vi "Construct Raw B-Scan.vi"(0 "1D Raw Data In":u16[](array[numeric]), 1 "Resample Array":i32[](array[numeric]), 2 "B-Scan Processed In":u32, 5 "B-Scans Per Transfer":u32, 9 "A-Scans Per B-Scan":u32, 11 "Points Per A-Scan":u32, 12 "Start Trim":u32, 13 "Stop Trim":u32, 14 "Scanning Parameters":T1={"Fast Axis Offset"=0.0, "Slow Axis Offset"=0.0, "Slow Axis Amp"=4.0, "Fast Axis Amp"=4.0, "Scan Pattern"=enum."Triangle Raster"} {"Fast Axis Amp" max=20 format="%#.2f"; "Slow Axis Amp" max=20 format="%#.2f"; "Slow Axis Offset" max=10 format="%#.2f"; "Fast Axis Offset" max=10 format="%#.2f"}) -> (3 "B-Scan Processed Out":u32, 4 "B-Scan In":u16[][][](array[numeric]), 10 "A-Scan Size":i32)   [LabVIEW 2015, in "Intensity Processing.lvclass"]
uses:
  Intensity/Intensity Processing.lvclass
  Galvo/Scanning Cluster.ctl
  Galvo/Galvo.lvclass
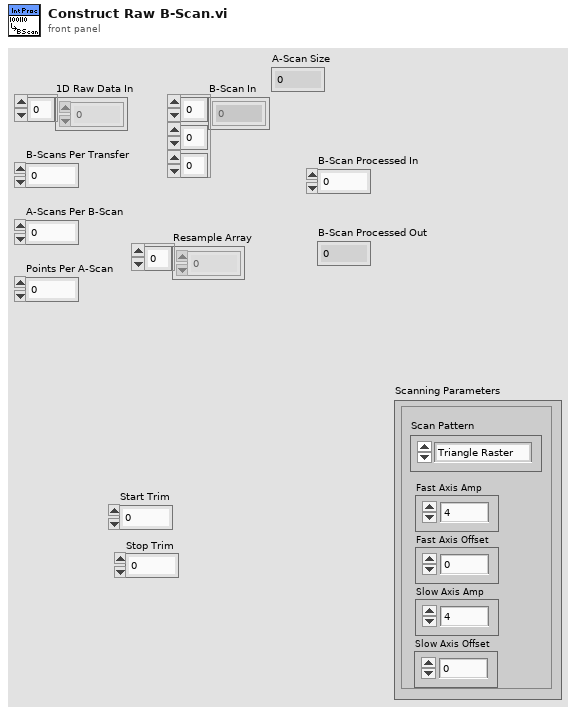
[diagram p1: front panel]
types:
  T1 = typedef "Galvo.lvclass/Scanning Cluster.ctl" = cluster{"Fast Axis Offset":sgl, "Slow Axis Offset":sgl, "Slow Axis Amp":sgl, "Fast Axis Amp":sgl, "Scan Pattern":enum16{"Raster", "Triangle Raster", "Sinusoid Raster"}}
  T2 = enum16{"Raster", "Triangle Raster", "Sinusoid Raster"}
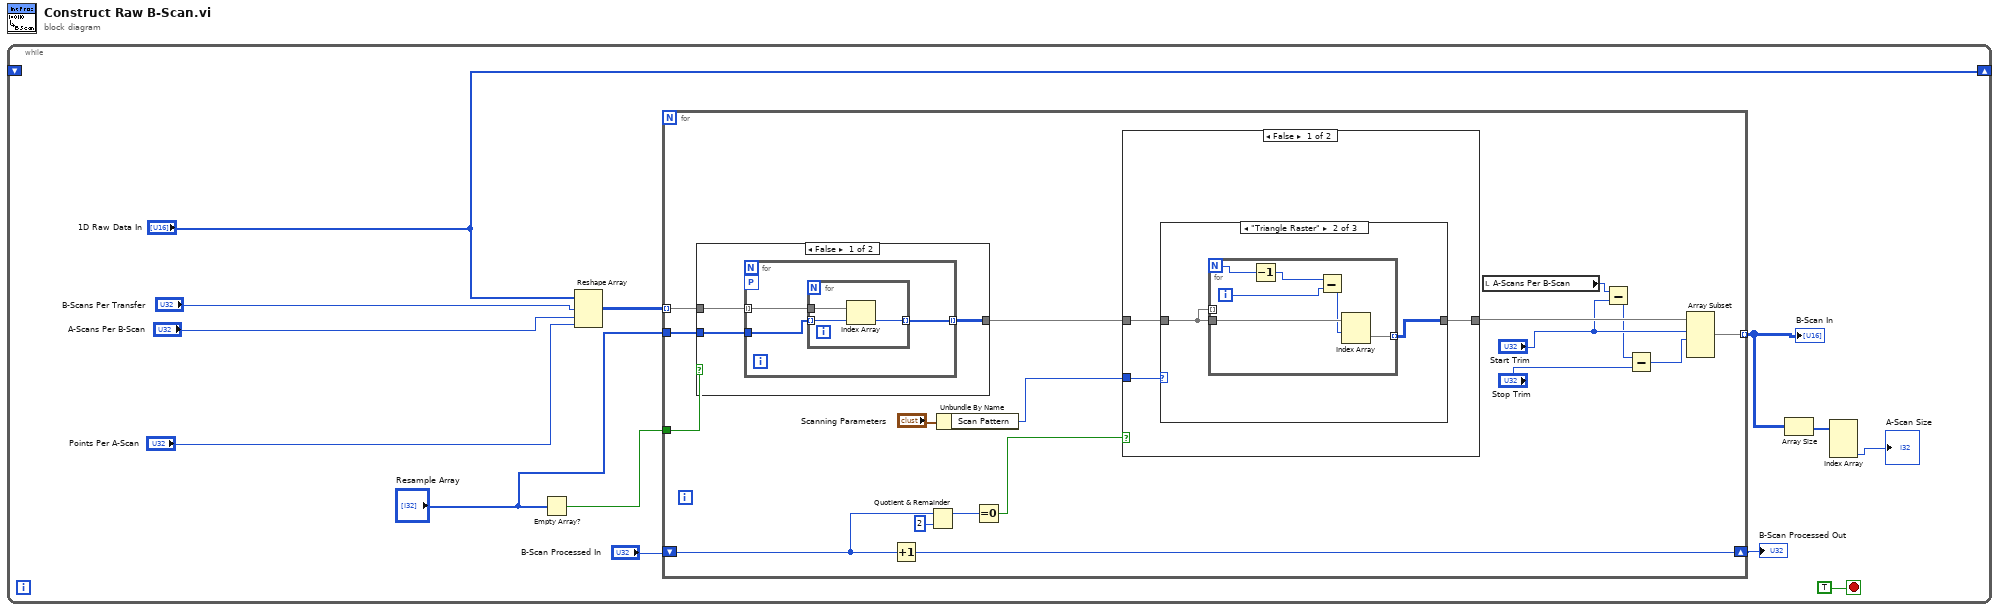
[diagram p0: block diagram]
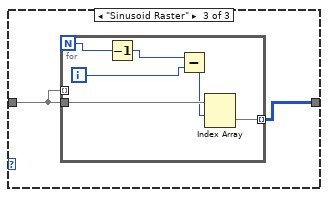
[diagram p3: hidden frame]
diagram:
  n1 = while {
    shift-right: ["1D Raw Data In"] -> _
    shift-left: _ -> [_]
    stop <- TRUE stop-if-true
    n2 = Empty Array?(array="Resample Array") -> (empty?=w8:bool)
    n3 = Reshape Array("1D Raw Data In", "B-Scans Per Transfer", "A-Scans Per B-Scan", "Points Per A-Scan") -> (w10:u16[][][])
    n4 = for {
      tunnel: w10 -> [w31] mode=indexing
      tunnel: "Resample Array" -> [w30]
      tunnel: w8 -> [w29]
      shift-right: [w24] -> w6
      shift-left: "B-Scan Processed In" -> [w25]
      tunnel: [w16] -> w3 mode=indexing
      n5 = case shown="False" w29 {
        tunnel: w31 -> [w55 w62]
        tunnel: [w54 w62] -> w27
        tunnel: w30 -> [w53 _]
        frame False {
          n6 = for {
            tunnel: w55 -> [w58] mode=indexing
            tunnel: [w57] -> w54 mode=indexing
            tunnel: w53 -> [w56]
            workers-P: _ -> [_]
            n7 = for {
              tunnel: w58 -> [w61]
              tunnel: w56 -> [w60] mode=indexing
              tunnel: [w59] -> w57 mode=indexing
              n8 = Index Array(array=w61, index=w60) -> (element=w59:u16)
            }
          }
        }
        frame True {
        }
      }
      n9 = Increment(x=w25) -> (x+1=w24:u32)
      n10 = Quotient & Remainder(x=w25, y=u32 2) -> (x-y*floor(x/y)=w23:u32)  [unwired: 1 out]
      n11 = Unbundle By Name("Scanning Parameters") -> ("Scan Pattern"=w14:T2)
      n12 = Equal To 0?(x=w23) -> (x = 0?=w26:bool)
      n13 = case shown="False" w26 {
        tunnel: w27 -> [w34 w52]
        tunnel: [w32 w52] -> w22
        tunnel: w14 -> [w33 _]
        frame False {
          n14 = case shown="\"Triangle Raster\"" w33 {
            tunnel: w34 -> [w35 w37 w45]
            tunnel: [w35 w36 w44] -> w32
            frame "Raster", Default {
            }
            frame "Triangle Raster" {
              n15 = for {
                N -> [w41]
                tunnel: w37 -> [w43]
                tunnel: [w42] -> w36 mode=indexing
                tunnel: w37 -> [_] mode=indexing
                i -> [w38]
                n16 = Decrement(x=w41) -> (x-1=w39:i32)
                n17 = Subtract(x=w39, y=w38) -> (x-y=w40:i32)
                n18 = Index Array(array=w43, index (row)=w40) -> (element=w42:u16[])  [unwired: 1 in]
              }
            }
            frame "Sinusoid Raster" {
              n19 = for {
                N -> [w49]
                tunnel: w45 -> [w51]
                tunnel: [w50] -> w44 mode=indexing
                tunnel: w45 -> [_] mode=indexing
                i -> [w46]
                n20 = Decrement(x=w49) -> (x-1=w47:i32)
                n21 = Subtract(x=w47, y=w46) -> (x-y=w48:i32)
                n22 = Index Array(array=w51, index (row)=w48) -> (element=w50:u16[])  [unwired: 1 in]
              }
            }
          }
        }
        frame True {
        }
      }
      n23 = local read "A-Scans Per B-Scan"() -> (w21:u32)
      n24 = Subtract(x=w21, y="Start Trim") -> (x-y=w19:u32)
      n25 = Subtract(x=w19, y="Stop Trim") -> (x-y=w17:u32)
      n26 = Array Subset(array=w22, index (row)="Start Trim", length (row)=w17) -> (w16:u16[][])  [unwired: 2 in]
    }
    "B-Scan Processed Out" <- w6
    "B-Scan In" <- w3
    n27 = Array Size(array=w3) -> (size(s)=w4:i32[])
    n28 = Index Array(array=w4) -> (element #3=→"A-Scan Size":i32)  [unwired: 3 in, 2 out]
  }
